vi "Lockin.Low Pass Filter.vi"(8 "error in (no error)":errorcluster, 11 "DSP in":refnum<class "DSP.lvclass">) -> (0 "error out":errorcluster, 3 "DSP out":refnum<class "DSP.lvclass">)   [LabVIEW 2020, in "DSP.lvclass"]
uses:
  DSP.lvclass
  DSP.lvclass/DSP.ctl
panel:
  out "Waveforms in":T1
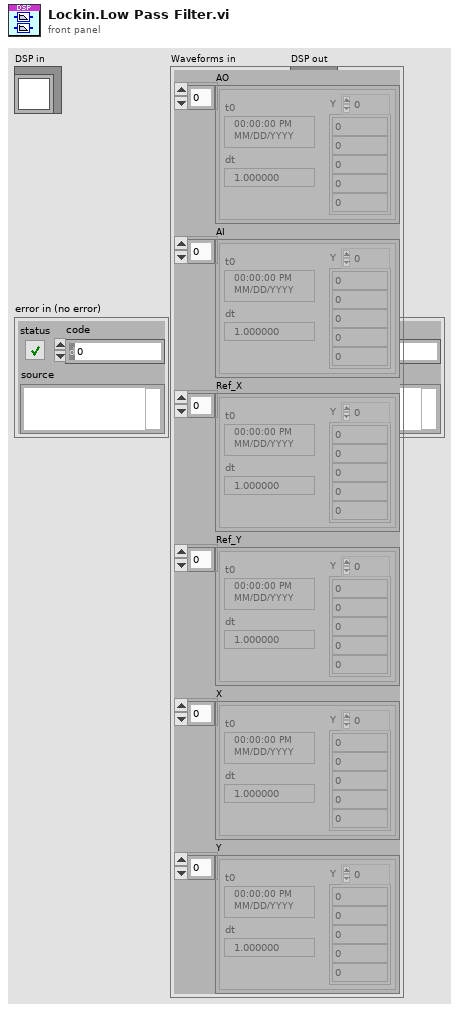
[diagram p1: front panel]
types:
  T1 = cluster{"AO":waveform(dbl)[], "AI":waveform(dbl)[], "Ref_X":waveform(dbl)[], "Ref_Y":waveform(dbl)[], "X":waveform(dbl)[], "Y":waveform(dbl)[]}
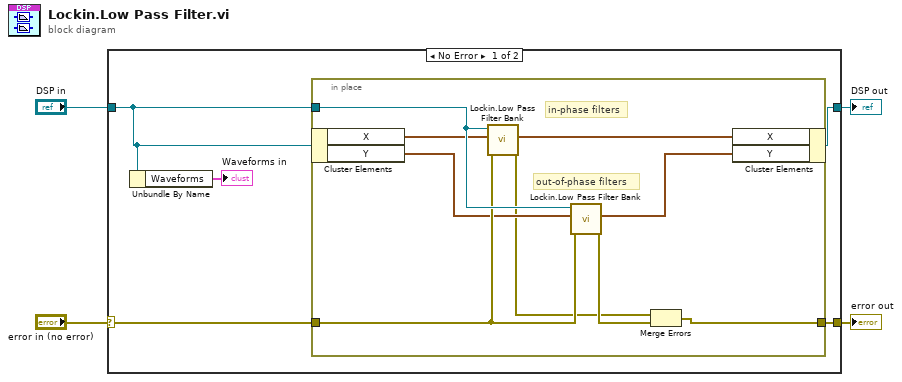
[diagram p0: block diagram]
diagram:
  n1 = case shown="No Error" "error in (no error)" {
    selector: "error in (no error)" -> [w8 w20]
    tunnel: [w9 w20] -> w4
    tunnel: [w7 w19] -> w3
    tunnel: "DSP in" -> [w6 w19]
    frame No Error {
      n2 = Unbundle By Name(w6) -> ("Waveforms"=→"Waveforms in":T1)
      n3 = in-place {
        in-place-border: [w18] -> w9
        in-place-border: w6 -> [w17]
        in-place-border: w8 -> [w16]
        # "out-of-phase filters"
        # "in-phase filters"
        n4 = in-place-cluster #1(w6) -> ("X"=w15:waveform(dbl)[], "Y"=w14:waveform(dbl)[])
        n5 = call "Lockin.Low Pass Filter Bank.vi"("error in (no error)"=w16, "WFms in"=w15, "DSP in"=w17) -> ("error out"=w12:errorcluster, "Wfms out"=w10:waveform(dbl)[])  [unwired: 7 in]
        n6 = call "Lockin.Low Pass Filter Bank.vi"("error in (no error)"=w16, "WFms in"=w14, "DSP in"=w17) -> ("error out"=w13:errorcluster, "Wfms out"=w11:waveform(dbl)[])  [unwired: 7 in]
        n7 = Merge Errors(w12, w13) -> (w18:errorcluster)
        n8 = in-place-cluster #1("X"=w10, "Y"=w11) -> (w7:refnum<class "DSP.lvclass">)
      }
    }
    frame Error {
    }
  }
  "error out" <- w4
  "DSP out" <- w3
